vi "Indentify line text box pos.vi"(8 "error in (no error)":errorcluster, 9 "text":string, 10 "PlotAreaBounds":T2, 11 "Coords":T3) -> (0 "error out":errorcluster, 3 "rect":T1)   [LabVIEW 2021, in "RocketPlot.lvlib"]
uses:
  RocketPlot.lvlib
  <vilib>/Utility/miscctls.llb/LVPoint32TypeDef.ctl
  <vilib>/Utility/miscctls.llb/LVRectTypeDef.ctl
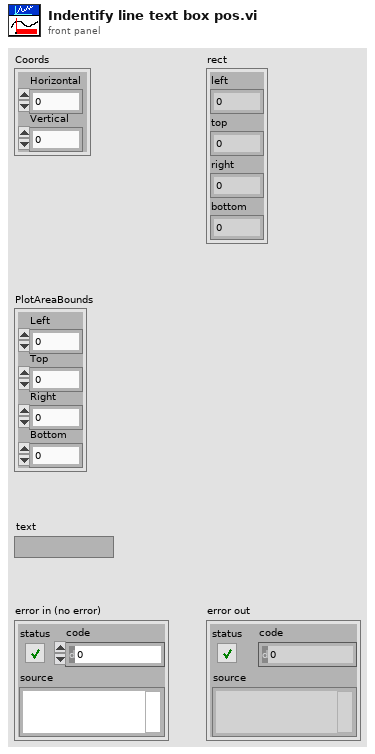
[diagram p1: front panel]
types:
  T1 = cluster{"left":i16, "top":i16, "right":i16, "bottom":i16}
  T2 = typedef "LVRectTypeDef.ctl" = cluster{"Left":i16, "Top":i16, "Right":i16, "Bottom":i16}
  T3 = typedef "LVPoint32TypeDef.ctl" = cluster{"Horizontal":i32, "Vertical":i32}
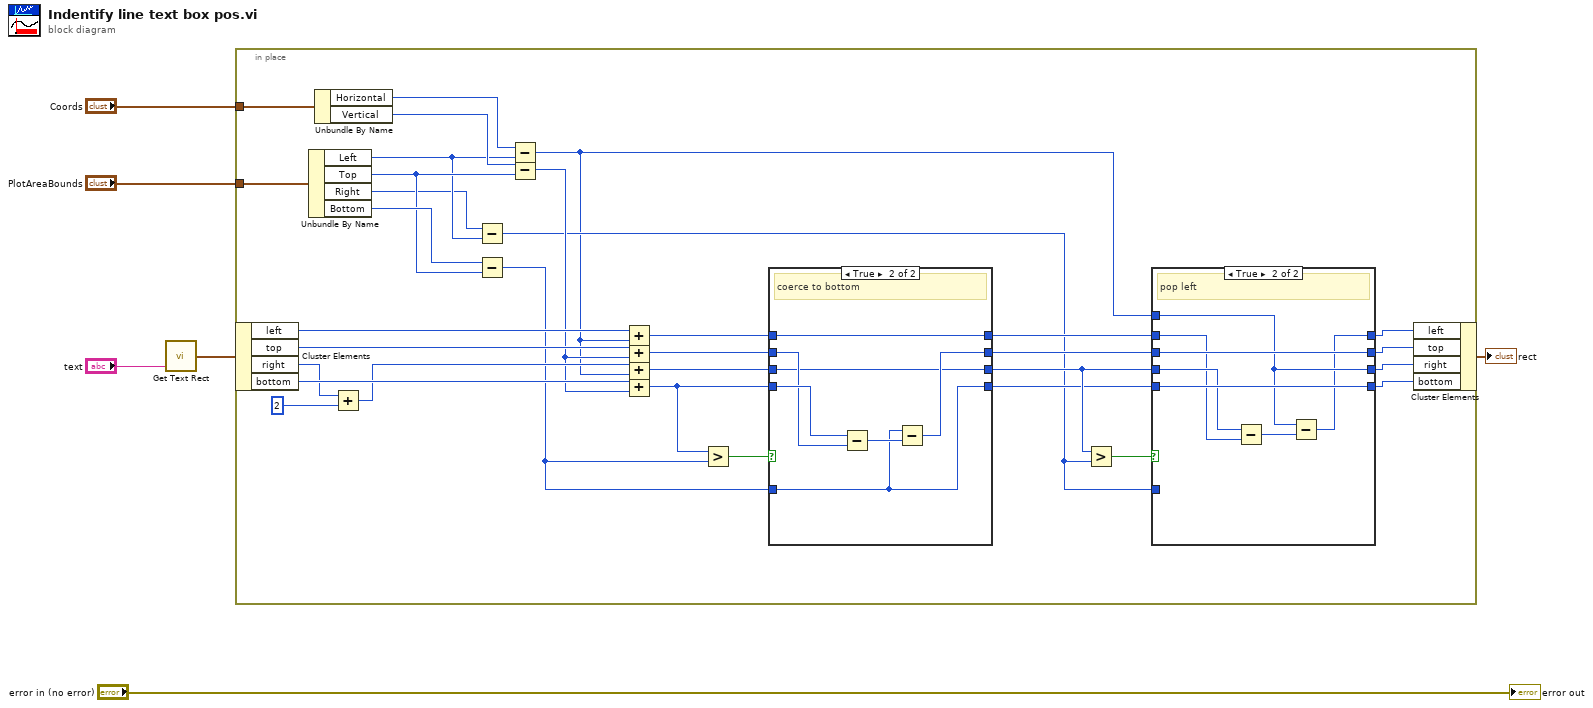
[diagram p0: block diagram]
diagram:
  n1 = call <vilib>:"Get Text Rect.vi"("text"="text") -> ("rect"=w5:T1)  [unwired: 8 in]
  n2 = in-place {
    in-place-border: "Coords" -> [w36]
    in-place-border: "PlotAreaBounds" -> [w37]
    n3 = in-place-cluster #1(w5) -> ("left"=w32:i16, "top"=w33:i16, "right"=w26:i16, "bottom"=w27:i16)
    n4 = Unbundle By Name(w37) -> ("Left"=w8:i16, "Top"=w20:i16, "Right"=w7:i16, "Bottom"=w22:i16)
    n5 = Unbundle By Name(w36) -> ("Horizontal"=w35:i32, "Vertical"=w34:i32)
    n6 = Add(x=w26, y=i16 2) -> (x+y=w25:i16)
    n7 = Subtract(x=w7, y=w8) -> (x-y=w10:i16)
    n8 = Subtract(x=w22, y=w20) -> (x-y=w21:i16)
    n9 = Subtract(x=w35, y=w8) -> (x-y=w9:i32)
    n10 = Subtract(x=w34, y=w20) -> (x-y=w24:i32)
    n11 = Add(x=w32, y=w9) -> (x+y=w30:i32)
    n12 = Add(x=w33, y=w24) -> (x+y=w29:i32)
    n13 = Add(x=w25, y=w9) -> (x+y=w28:i32)
    n14 = Add(x=w27, y=w24) -> (x+y=w23:i32)
    n15 = Greater?(x=w23, y=w21) -> (0:w31:bool)
    n16 = case shown="True" w31 {
      tunnel: w30 -> [w53 w56]
      tunnel: [w53 w56] -> w19
      tunnel: w29 -> [w52 w59]
      tunnel: [w52 w57] -> w18
      tunnel: w28 -> [w51 w55]
      tunnel: [w51 w55] -> w17
      tunnel: w23 -> [w50 w60]
      tunnel: [w50 w54] -> w16
      tunnel: w21 -> [_ w54]
      frame False {
      }
      frame True {
        # "coerce to bottom"
        n17 = Subtract(x=w60, y=w59) -> (x-y=w58:i32)
        n18 = Subtract(x=w54, y=w58) -> (x-y=w57:i32)
      }
    }
    n19 = Greater?(x=w17, y=w10) -> (0:w15:bool)
    n20 = case shown="True" w15 {
      tunnel: w19 -> [w42 w46]
      tunnel: [w42 w43] -> w14
      tunnel: w18 -> [w41 w49]
      tunnel: [w41 w49] -> w13
      tunnel: w17 -> [w40 w47]
      tunnel: [w40 w45] -> w12
      tunnel: w16 -> [w39 w48]
      tunnel: [w39 w48] -> w11
      tunnel: w10 -> [_ _]
      tunnel: w9 -> [_ w45]
      frame False {
      }
      frame True {
        # "pop left"
        n21 = Subtract(x=w47, y=w46) -> (x-y=w44:i32)
        n22 = Subtract(x=w45, y=w44) -> (x-y=w43:i32)
      }
    }
    n23 = in-place-cluster #1("left"=w14, "top"=w13, "right"=w12, "bottom"=w11) -> (→"rect":T1)
  }
  "error out" <- "error in (no error)"
